vi "TurnScheme.vi"(3 "Real Matrix":T1) -> (1 "Array":bool[][](array[boolean]))   [LabVIEW 2018]
doc: "Позволяет перевести любую матрицу со значениями 0 и 1 в boolean массив"
uses:
  <vilib>/Analysis/Matrix/Datatypes/RealMatrix.ctl
  <vilib>/Analysis/Matrix/Numeric/Conversions/Matrix To Array - RM.vi
  <vilib>/Analysis/Matrix/NI_Matrix.lvlib
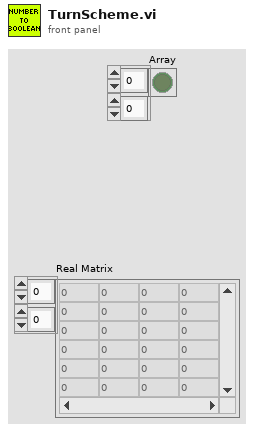
[diagram p1: front panel]
types:
  T1 = typedef "NI_Matrix.lvlib/RealMatrix.ctl" = dbl[][]
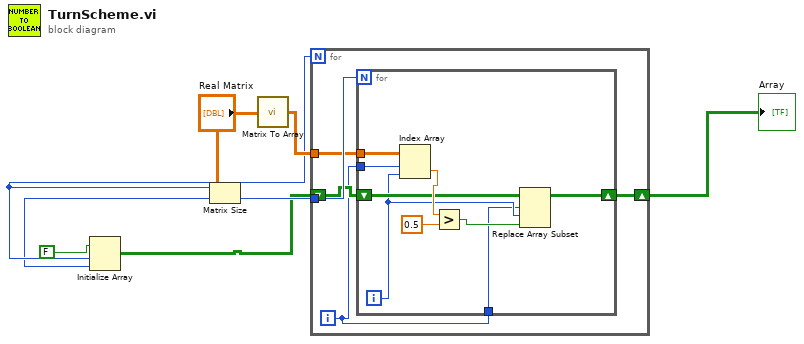
[diagram p0: block diagram]
diagram:
  n1 = Matrix Size(0:"Real Matrix") -> (1:w5:i32, 2:w4:i32)
  n2 = Initialize Array(FALSE, w5, w4) -> (w2:bool[][])
  n3 = call-poly <vilib>:"Matrix To Array.vi"("Real Matrix"="Real Matrix") -> ("Real 2D Array"=w6:dbl[][])
  n4 = for {
    N: w5 -> [_]
    tunnel: w4 -> [w12]
    tunnel: w6 -> [w11]
    shift-right: [w8] -> w1
    shift-left: w2 -> [w10]
    i -> [w9]
    n5 = for {
      N: w12 -> [_]
      tunnel: w11 -> [w21]
      tunnel: w9 -> [w20]
      tunnel: w9 -> [w14]
      shift-right: [w13] -> w8
      shift-left: w10 -> [w17]
      i -> [w15]
      n6 = Index Array(array=w21, index (row)=w20, index (col)=w15) -> (element=w19:dbl)
      n7 = Greater?(x=w19, y=0.5) -> (0:w16:bool)
      n8 = Replace Array Subset(array=w17, new element=w16, index (row)=w14, index (col)=w15) -> (w13:bool[][])
    }
  }
  "Array" <- w1
